vi "Day 15 Waveform & format.vi"() -> ()   [LabVIEW 2026]
panel:
  out "Formatted Unit Readout String":string
  out "output waveform":waveform(dbl)
  out "Waveform Graph":waveform(dbl)(graph)
  out "Array":dbl[](array[numeric])
  # "Build a waveform from an array and display it on a graph."
  # "Format a numeric result into a string with three decimals and a unit"
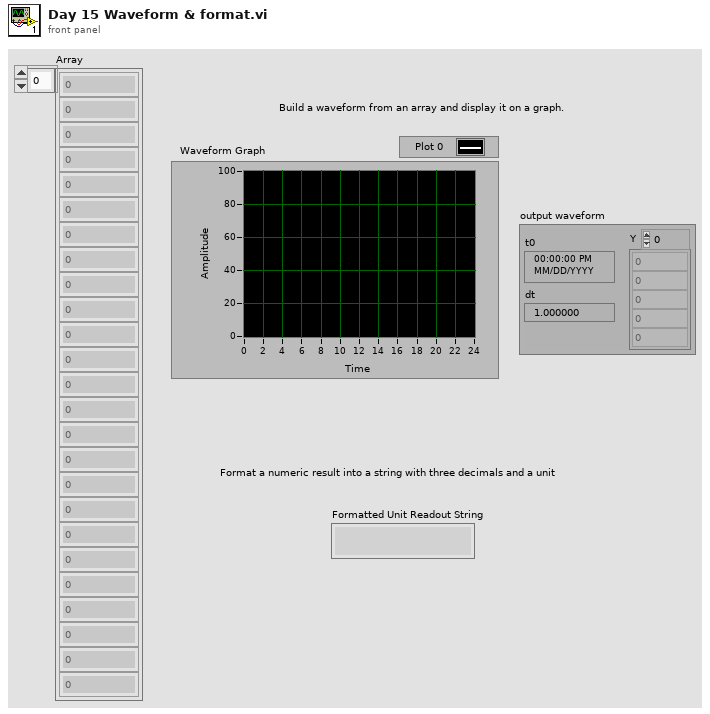
[diagram p1: front panel]
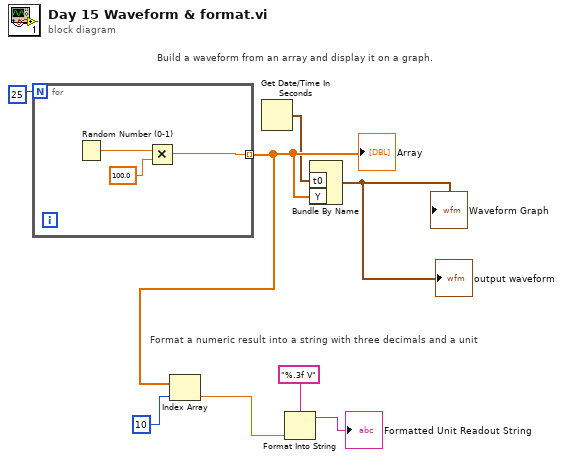
[diagram p0: block diagram]
diagram:
  # "Format a numeric result into a string with three decimals and a unit"
  # "Build a waveform from an array and display it on a graph."
  n1 = for {
    N: 25 -> [_]
    tunnel: [w9] -> w2 mode=indexing
    n2 = Random Number (0-1)() -> (number: 0 to 1=w11:dbl)
    n3 = Multiply(x=w11, y=100.0) -> (x*y=w9:dbl)
  }
  "Array" <- w2
  n4 = Index Array "Index Array"(array=w2, index=10) -> (element=w5:dbl)
  n5 = Get Date/Time In Seconds() -> (seconds since 1Jan1904=w1:timestamp)
  n6 = Format Into String(format string="%.3f V", w5) -> (resulting string=→"Formatted Unit Readout String":string)  [unwired: 2 in, 1 out]
  n7 = Bundle By Name("t0"=w1, "Y"=w2) -> (→"Waveform Graph" →"output waveform":waveform(dbl))  [unwired: 1 in]
